vi "WPI_RobotDriveTankDrive2.vi"(8 "error in (no error)":errorcluster, 9 "Right axis value":dbl, 10 "Left axis value":dbl, 11 "RobotDriveDevRef":T1={"DevStatus"={"status"=FALSE, "code"=0, "source"=""}, "Motors[]"=[], "Square Inputs"=FALSE, "Max Output"=1.0, "Isochronous"=FALSE}) -> (0 "error out":errorcluster, 3 "RobotDriveDevRef":T1={"DevStatus"={"status"=FALSE, "code"=0, "source"=""}, "Motors[]"=[], "Square Inputs"=FALSE, "Max Output"=1.0, "Isochronous"=FALSE})   [LabVIEW 2012]
doc: "Configures the motors for tank driving. Tank driving uses two joysticks where the y-axis values of each joystick specify the power to apply to the motors on either side of the robot.\n\nThis software is licensed. Open the labview\\readme\\WPI Robotics Library Open Source License.txt file for more information."
uses:
  <vilib>/Rock Robotics/WPI/RobotDrive/WPI_RobotDriveDevRef.ctl
  <vilib>/Rock Robotics/WPI/MotorControl/WPI_MotorControlDeviceRef.ctl
  <vilib>/Rock Robotics/SystemInterfaces/Typedef/FPGA_TypedefDigitalModule.ctl
  <vilib>/Rock Robotics/SystemInterfaces/DIO/FPGA_DIOPWMChannel.ctl
  <vilib>/Rock Robotics/WPI/PWM/WPI_PWMDeadband.ctl
  <vilib>/Rock Robotics/WPI/CAN/Jaguar/SubVIs/WPI_CANJaguar_ControlMode.ctl
  <vilib>/Rock Robotics/WPI/PWM/WPI_PWMTransform_ConPane.ctl
  <vilib>/Rock Robotics/SystemInterfaces/NetworkCommunication/NetComm_UsageReport_ResourceType.ctl
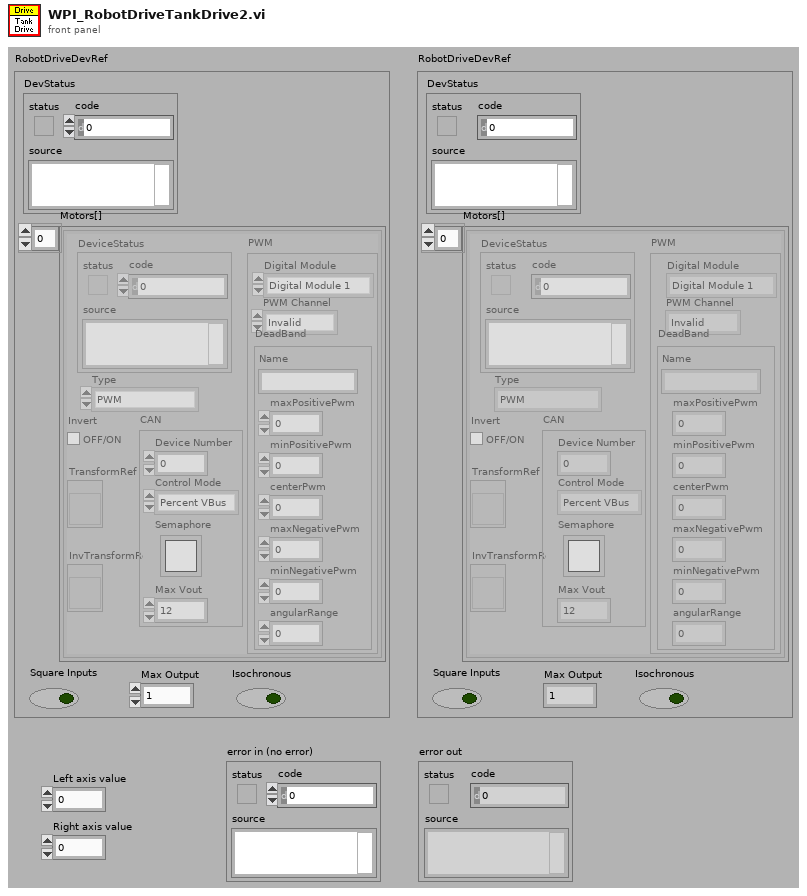
[diagram p1: front panel]
types:
  T1 = typedef "WPI_RobotDriveDevRef.ctl" = cluster{"DevStatus":errorcluster, "Motors[]":T2[], "Square Inputs":bool, "Max Output":dbl, "Isochronous":bool}
  T2 = typedef "WPI_MotorControlDeviceRef.ctl" = cluster{"DeviceStatus":errorcluster, "Type":enum16{"PWM", "CAN"}, "PWM":cluster{"Digital Module":T3, "PWM Channel":T4, "DeadBand":T5}, "CAN":cluster{"Device Number":u8, "Control Mode":T6, "Semaphore":T7, "Max Vout":dbl}, "Invert":bool, "TransformRef":T8, "InvTransformRef":T8}
  T3 = typedef "FPGA_TypedefDigitalModule.ctl" = enum16{"Digital Module 1", "Digital Module 2"}
  T4 = typedef "FPGA_DIOPWMChannel.ctl" = enum8{"PWM 1", "PWM 2", "PWM 3", "PWM 4", "PWM 5", "PWM 6", "PWM 7", "PWM 8", "PWM 9", "PWM 10", "Invalid"}
  T5 = typedef "WPI_PWMDeadband.ctl" = cluster{"Name":string, "maxPositivePwm":i32, "minPositivePwm":i32, "centerPwm":i32, "maxNegativePwm":i32, "minNegativePwm":i32, "angularRange":u16}
  T6 = typedef "WPI_CANJaguar_ControlMode.ctl" = enum8{"Percent VBus", "Current", "Speed", "Position", "Voltage"}
  T7 = typedef "Semaphore RefNum" = refnum<k1>
  T8 = typedef "WPI_PWMTransform_ConPane.ctl" = refnum<vi>
  T9 = typedef "NetComm_UsageReport_ResourceType.ctl" = enum8{"Controller", "Module", "Language", "CANPlugin", "Accelerometer", "ADXL345", "AnalogChannel", "AnalogTrigger", "AnalogTriggerOutput", "CANJaguar", "Compressor", "Counter", "Dashboard", "DigitalInput", "DigitalOutput", "DriverStationCIO", "DriverStationEIO", "DriverStationLCD", "Encoder", "GearTooth", "Gyro", "I2C", "Framework", "Jaguar", "Joystick", "Kinect", "KinectStick", "PIDController", "Preferences", "PWM", "Relay", "RobotDrive", "SerialPort", "Servo", "Solenoid", "SPI", "Task", "Ultrasonic", "Victor", "Button", "Command", "AxisCamera", "PCVideoServer", "SmartDashboard", "Talon", "HiTechnicColorSensor", "HiTechnicAccel", "HiTechnicCompass", "SRF08"}
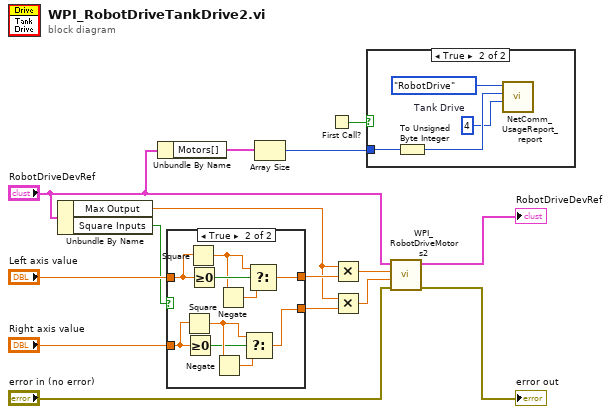
[diagram p0: block diagram]
diagram:
  n1 = Unbundle By Name("RobotDriveDevRef") -> ("Max Output"=w7:dbl, "Square Inputs"=w11:bool)
  n2 = Unbundle By Name("RobotDriveDevRef") -> ("Motors[]"=w3:T2[])
  n3 = case shown="True" w11 {
    tunnel: "Left axis value" -> [w17 w27]
    tunnel: [w17 w23] -> w13
    tunnel: [w16 w19] -> w9
    tunnel: "Right axis value" -> [w16 w18]
    frame False {
    }
    frame True {
      n4 = Square(x=w18) -> (x^2=w21:dbl)
      n5 = Greater Or Equal To 0?(x=w18) -> (x >= 0?=w20:bool)
      n6 = Square(x=w27) -> (x^2=w25:dbl)
      n7 = Greater Or Equal To 0?(x=w27) -> (x >= 0?=w26:bool)
      n8 = Negate(x=w21) -> (-x=w22:dbl)
      n9 = Negate(x=w25) -> (-x=w24:dbl)
      n10 = Select(t=w21, s=w20, f=w22) -> (s? t:f=w19:dbl)
      n11 = Select(t=w25, s=w26, f=w24) -> (s? t:f=w23:dbl)
    }
  }
  n12 = Array Size(array=w3) -> (size(s)=w2:i32)
  n13 = First Call?() -> (First Call?: T/F=w4:bool)
  n14 = Multiply(x=w7, y=w13) -> (x*y=w10:dbl)
  n15 = Multiply(x=w7, y=w9) -> (x*y=w8:dbl)
  n16 = case shown="True" w4 {
    tunnel: w2 -> [_ w30]
    frame False {
    }
    frame True {
      w28 = u8 4  # Tank Drive
      n17 = To Unsigned Byte Integer(number=w30) -> (unsigned 8bit integer=w29:u8)
      n18 = call <vilib>:"NetComm_UsageReport_report.vi"("Context"=w28, "Instance Number"=w29, "Resource Type"=NetComm_UsageReport_ResourceType."RobotDrive") -> ()  [unwired: 9 in]
    }
  }
  n19 = call "WPI_RobotDriveMotors2.vi"("error in (no error)"="error in (no error)", "RightSpeed"=w8, "LeftSpeed"=w10, "RobotDriveDevRef"="RobotDriveDevRef") -> ("error out"=→"error out":errorcluster, "RobotDriveDevRef"=→"RobotDriveDevRef":T1)  [unwired: 6 in]
